vi "Image to SGL Array.vi"(7 "Optional Rectangle":i32[](array[numeric]), 8 "error in (no error)":errorcluster, 11 "Image":T1) -> (0 "error out":errorcluster, 1 "Y Resolution":i32, 2 "X Resolution":i32, 3 "Image Pixels (Float)":sgl[][](array[numeric]))   [LabVIEW 2021, in "Image.lvlib"]
uses:
  Image.lvlib
  <vilib>/vision/Image Controls.llb/IMAQ Image.ctl
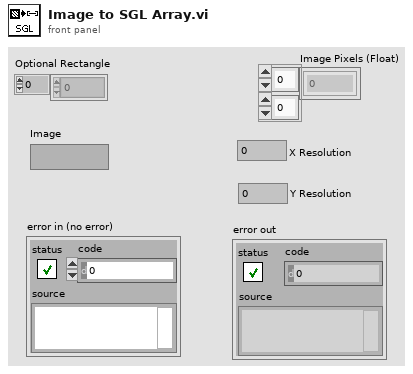
[diagram p1: front panel]
types:
  T1 = typedef "IMAQ Image.ctl" = refnum<image>
  T2 = typedef "Image Type" = u32
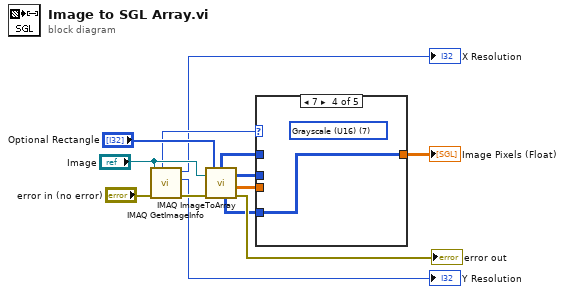
[diagram p0: block diagram]
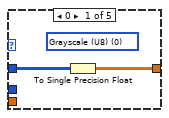
[diagram p2: hidden frame]
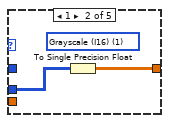
[diagram p3: hidden frame]
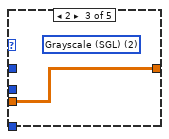
[diagram p4: hidden frame]
diagram:
  n1 = call "IMAQ GetImageInfo"("error in (no error)"="error in (no error)", "Image"="Image") -> ("error out"=w12:errorcluster, "Y Resolution"=→"Y Resolution":i32, "X Resolution"=→"X Resolution":i32, "Image Type"=w9:T2)  [unwired: 2 in, 4 out]
  n2 = call "IMAQ ImageToArray"("error in (no error)"=w12, "Optional Rectangle"="Optional Rectangle", "Image"="Image") -> ("Image Pixels (U16)"=w3:u16[][], "Image Pixels (Float)"=w6:sgl[][], "error out"=→"error out":errorcluster, "Image Pixels (U8)"=w8:u8[][], "Image Pixels (I16)"=w7:i16[][])  [unwired: 1 in]
  n3 = case shown="7" w9 {
    tunnel: w8 -> [w15 _ _ _ _]
    tunnel: [w14 w17 w18 w19 _] -> w4
    tunnel: w7 -> [_ w16 _ _ _]
    tunnel: w6 -> [_ _ w18 _ _]
    tunnel: w3 -> [_ _ _ w19 _]
    frame 0 {
      (unwired) T2 0 items=["Grayscale (U8)", "Grayscale (I16)", "Grayscale (SGL)", "Complex (CSG)", "RGB (U32)", "HSL (U32)", "RGB (U64)", "Grayscale (U16)"] ("Image Type")
      n4 = To Single Precision Float(number=w15) -> (single precision float=w14:sgl[][])
    }
    frame 1 {
      (unwired) T2 1 items=["Grayscale (U8)", "Grayscale (I16)", "Grayscale (SGL)", "Complex (CSG)", "RGB (U32)", "HSL (U32)", "RGB (U64)", "Grayscale (U16)"] ("Image Type")
      n5 = To Single Precision Float(number=w16) -> (single precision float=w17:sgl[][])
    }
    frame 2 {
      (unwired) T2 2 items=["Grayscale (U8)", "Grayscale (I16)", "Grayscale (SGL)", "Complex (CSG)", "RGB (U32)", "HSL (U32)", "RGB (U64)", "Grayscale (U16)"] ("Image Type")
    }
    frame 7 {
      (unwired) T2 7 items=["Grayscale (U8)", "Grayscale (I16)", "Grayscale (SGL)", "Complex (CSG)", "RGB (U32)", "HSL (U32)", "RGB (U64)", "Grayscale (U16)"] ("Image Type")
    }
    frame 3, Default {
    }
  }
  "Image Pixels (Float)" <- w4
